vi "Stepper -- V3.vi"() -> ()   [LabVIEW 2018]
doc: "Use this template to build a producer/consumer design pattern with events to produce queue items. Use this design pattern instead of the User Interface Event Handler pattern for user interfaces when you want to execute code asynchronously in response to an event without slowing the user interface responsiveness."
uses:
  stepper motor state.ctl
  stepper graphics internal event.ctl
  stepper graphics action.ctl
  stepper graphics internal state.ctl
  stepper driver action.ctl
  publisher action.ctl
  slider action.ctl
  stepper driver -- BLM.vi
  stepper driver -- IMS.vi
panel:
  in  "Tab Control":enum32{"main", "init&stuff", "ignore"}(tab)
  in  "speed":i32=4003
  in  "stepper state":T1=enum."stopped"
  in  "set angle":dbl(slide)=-10.106382978723403 scale=-56.0..55.0 scale format="%^#6_6g"
  in  "XY Graph":cluster{dbl[], dbl[]}[](graph)=[{[-0.30000000000000004, -0.23550000000000004, -0.17100000000000004, -0.10650000000000004, -0.04200000000000004, 0.022499999999999964, 0.08699999999999997, 0.15149999999999997, 0.21599999999999997, 0.28049999999999997, 0.345, 0.4095, 0.474, 0.5385, 0.603, 0.6675, 0.732, 0.7965, 0.861, 0.9255], [0.0, 0.0, 0.0, 0.0, 0.0, 0.0, 0.0, 0.0, 0.0, 0.0, 0.0, 0.0, 0.0, 0.0, 0.0, 0.0, 0.0, 0.0, 0.0, 0.0]}, {[-0.29607463230851366, -0.23241858636218324, -0.1687625404158528, -0.10510649446952239, -0.04145044852319196, 0.02220559742313849, 0.08586164336946889, 0.14951768931579928, 0.21317373526212974, 0.2768297812084602, 0.34048582715479064, 0.404141873101121, 0.46779791904745144, 0.531453964993782, 0.5951100109401122, 0.6587660568864426, 0.7224221028327731, 0.7860781487791035, 0.849734194725434, 0.9133902406717644], [0.048371604308503874, 0.03797170938217554, 0.02757181445584721, 0.01717191952951888, 0.006772024603190548, -0.0036278703231377857, -0.014027765249466112, -0.024427660175794452, -0.03482755510212278, -0.045227450028451105, -0.055627344954779445, -0.06602723988110777, -0.0764271348074361, -0.08682702973376444, -0.09722692466009278, -0.10762681958642109, -0.11802671451274943, -0.12842660943907777, -0.13882650436540608, -0.14922639929173442]}, {[1.0, 0.9980267284282716, 0.9921147013144779, 0.9822872507286887, 0.9685831611286311, 0.9510565162951535, 0.9297764858882513, 0.9048270524660195, 0.8763066800438636, 0.8443279255020151, 0.8090169943749475, 0.7705132427757891, 0.7289686274214116, 0.6845471059286886, 0.6374239897486896, 0.587785252292473, 0.5358267949789965, 0.48175367410171516, 0.42577929156507266, 0.36812455268467786, 0.30901699437494745, 0.24868988716485474, 0.18738131458572452, 0.12533323356430426, 0.0627905195293133, -1.6081428723391245e-16, -0.0627905195293134, -0.12533323356430437, -0.18738131458572482, -0.24868988716485485, -0.30901699437494756, -0.368124552684678, -0.4257792915650727, -0.48175367410171543, -0.5358267949789969, -0.587785252292473, -0.6374239897486897, -0.6845471059286887, -0.7289686274214117, -0.7705132427757894, -0.8090169943749473, -0.8443279255020151, -0.8763066800438636, -0.9048270524660196, -0.9297764858882515, -0.9510565162951536, -0.9685831611286311, -0.9822872507286887, -0.9921147013144779, -0.9980267284282716, -1.0, -0.9980267284282716, -0.9921147013144779, -0.9822872507286886, -0.9685831611286311, -0.9510565162951535, -0.9297764858882512, -0.9048270524660195, -0.8763066800438635, -0.844327925502015, -0.8090169943749472, -0.770513242775789, -0.7289686274214116, -0.6845471059286886, -0.6374239897486895, -0.5877852522924732, -0.5358267949789963, -0.48175367410171527, -0.42577929156507216, -0.3681245526846778, -0.30901699437494756, -0.24868988716485443, -0.18738131458572463, -0.12533323356430373, -0.06279051952931321, -1.836909530733566e-16, 0.06279051952931372, 0.12533323356430423, 0.18738131458572513, 0.24868988716485493, 0.30901699437494723, 0.36812455268467825, 0.4257792915650726, 0.4817536741017157, 0.5358267949789968, 0.5877852522924737, 0.63742398974869, 0.6845471059286886, 0.7289686274214119, 0.7705132427757894, 0.8090169943749478, 0.8443279255020153, 0.8763066800438636, 0.9048270524660197, 0.9297764858882515, 0.9510565162951538, 0.9685831611286312, 0.9822872507286887, 0.9921147013144779, 0.9980267284282716], [0.0, 0.06279051952931337, 0.12533323356430426, 0.18738131458572463, 0.2486898871648548, 0.3090169943749474, 0.368124552684678, 0.4257792915650727, 0.4817536741017153, 0.5358267949789967, 0.5877852522924731, 0.6374239897486897, 0.6845471059286887, 0.7289686274214116, 0.7705132427757893, 0.8090169943749475, 0.8443279255020151, 0.8763066800438637, 0.9048270524660196, 0.9297764858882515, 0.9510565162951535, 0.9685831611286311, 0.9822872507286887, 0.9921147013144779, 0.9980267284282716, 1.0, 0.9980267284282716, 0.9921147013144778, 0.9822872507286886, 0.9685831611286311, 0.9510565162951535, 0.9297764858882513, 0.9048270524660195, 0.8763066800438635, 0.844327925502015, 0.8090169943749475, 0.7705132427757893, 0.7289686274214114, 0.6845471059286885, 0.6374239897486895, 0.5877852522924732, 0.5358267949789967, 0.4817536741017152, 0.4257792915650725, 0.36812455268467775, 0.3090169943749471, 0.24868988716485482, 0.18738131458572457, 0.1253332335643041, 0.06279051952931314, -3.216285744678249e-16, -0.06279051952931335, -0.12533323356430429, -0.18738131458572477, -0.24868988716485502, -0.30901699437494773, -0.3681245526846783, -0.42577929156507266, -0.4817536741017154, -0.5358267949789968, -0.5877852522924734, -0.63742398974869, -0.6845471059286887, -0.7289686274214116, -0.7705132427757894, -0.8090169943749473, -0.8443279255020153, -0.8763066800438636, -0.9048270524660198, -0.9297764858882515, -0.9510565162951535, -0.9685831611286312, -0.9822872507286887, -0.9921147013144779, -0.9980267284282716, -1.0, -0.9980267284282716, -0.9921147013144779, -0.9822872507286886, -0.9685831611286311, -0.9510565162951536, -0.9297764858882512, -0.9048270524660196, -0.8763066800438634, -0.844327925502015, -0.809016994374947, -0.770513242775789, -0.7289686274214116, -0.6845471059286883, -0.6374239897486896, -0.5877852522924726, -0.5358267949789963, -0.4817536741017153, -0.4257792915650722, -0.36812455268467786, -0.3090169943749468, -0.2486898871648545, -0.18738131458572468, -0.1253332335643038, -0.06279051952931326]}, {[0.1, 0.09980267284282716, 0.0992114701314478, 0.09822872507286888, 0.09685831611286311, 0.09510565162951536, 0.09297764858882514, 0.09048270524660196, 0.08763066800438636, 0.08443279255020152, 0.08090169943749476, 0.07705132427757892, 0.07289686274214116, 0.06845471059286887, 0.06374239897486897, 0.05877852522924731, 0.05358267949789966, 0.04817536741017152, 0.042577929156507266, 0.03681245526846779, 0.030901699437494747, 0.024868988716485477, 0.018738131458572452, 0.012533323356430426, 0.006279051952931331, -1.6081428723391246e-17, -0.0062790519529313405, -0.012533323356430438, -0.018738131458572484, -0.024868988716485487, -0.030901699437494757, -0.0368124552684678, -0.04257792915650727, -0.048175367410171546, -0.05358267949789969, -0.05877852522924731, -0.06374239897486898, -0.06845471059286888, -0.07289686274214117, -0.07705132427757894, -0.08090169943749474, -0.08443279255020152, -0.08763066800438636, -0.09048270524660196, -0.09297764858882515, -0.09510565162951537, -0.09685831611286311, -0.09822872507286888, -0.0992114701314478, -0.09980267284282716, -0.1, -0.09980267284282716, -0.0992114701314478, -0.09822872507286887, -0.09685831611286311, -0.09510565162951536, -0.09297764858882512, -0.09048270524660196, -0.08763066800438635, -0.0844327925502015, -0.08090169943749473, -0.07705132427757891, -0.07289686274214116, -0.06845471059286887, -0.06374239897486896, -0.05877852522924733, -0.05358267949789963, -0.04817536741017153, -0.04257792915650722, -0.036812455268467784, -0.030901699437494757, -0.024868988716485445, -0.018738131458572463, -0.012533323356430374, -0.006279051952931321, -1.836909530733566e-17, 0.006279051952931373, 0.012533323356430424, 0.018738131458572515, 0.024868988716485494, 0.030901699437494726, 0.036812455268467825, 0.042577929156507266, 0.048175367410171574, 0.05358267949789968, 0.05877852522924737, 0.063742398974869, 0.06845471059286887, 0.07289686274214119, 0.07705132427757894, 0.08090169943749478, 0.08443279255020153, 0.08763066800438636, 0.09048270524660197, 0.09297764858882515, 0.09510565162951538, 0.09685831611286312, 0.09822872507286888, 0.0992114701314478, 0.09980267284282716], [0.0, 0.006279051952931338, 0.012533323356430426, 0.018738131458572463, 0.02486898871648548, 0.03090169943749474, 0.0368124552684678, 0.04257792915650727, 0.04817536741017153, 0.05358267949789967, 0.058778525229247314, 0.06374239897486898, 0.06845471059286888, 0.07289686274214116, 0.07705132427757894, 0.08090169943749476, 0.08443279255020152, 0.08763066800438638, 0.09048270524660196, 0.09297764858882515, 0.09510565162951536, 0.09685831611286311, 0.09822872507286888, 0.0992114701314478, 0.09980267284282716, 0.1, 0.09980267284282716, 0.09921147013144778, 0.09822872507286887, 0.09685831611286311, 0.09510565162951536, 0.09297764858882514, 0.09048270524660196, 0.08763066800438635, 0.0844327925502015, 0.08090169943749476, 0.07705132427757894, 0.07289686274214115, 0.06845471059286885, 0.06374239897486896, 0.05877852522924733, 0.05358267949789967, 0.048175367410171525, 0.04257792915650725, 0.03681245526846778, 0.030901699437494712, 0.024868988716485484, 0.01873813145857246, 0.01253332335643041, 0.0062790519529313145, -3.216285744678249e-17, -0.006279051952931335, -0.01253332335643043, -0.018738131458572477, -0.024868988716485504, -0.030901699437494774, -0.03681245526846783, -0.042577929156507266, -0.04817536741017154, -0.05358267949789968, -0.05877852522924734, -0.063742398974869, -0.06845471059286888, -0.07289686274214116, -0.07705132427757894, -0.08090169943749474, -0.08443279255020153, -0.08763066800438636, -0.09048270524660199, -0.09297764858882515, -0.09510565162951536, -0.09685831611286312, -0.09822872507286888, -0.0992114701314478, -0.09980267284282716, -0.1, -0.09980267284282716, -0.0992114701314478, -0.09822872507286887, -0.09685831611286311, -0.09510565162951537, -0.09297764858882512, -0.09048270524660196, -0.08763066800438635, -0.0844327925502015, -0.0809016994374947, -0.07705132427757891, -0.07289686274214116, -0.06845471059286883, -0.06374239897486897, -0.05877852522924726, -0.05358267949789963, -0.04817536741017153, -0.042577929156507224, -0.03681245526846779, -0.03090169943749468, -0.02486898871648545, -0.01873813145857247, -0.012533323356430379, -0.006279051952931327]}, {[0.0, 0.0, 0.0, 0.0, 0.0, 0.0, 0.0, 0.0, 0.0, 0.0, 0.0, 0.0, 0.0, 0.0, 0.0, 0.0, 0.0, 0.0, 0.0, 0.0], [1.1, 1.135, 1.1700000000000002, 1.205, 1.24, 1.2750000000000001, 1.31, 1.345, 1.3800000000000001, 1.415, 1.4500000000000002, 1.485, 1.52, 1.5550000000000002, 1.59, 1.625, 1.6600000000000001, 1.695, 1.73, 1.7650000000000001]}, {[-0.09587131702242406, -0.09674287444990064, -0.09761443187737723, -0.0984859893048538, -0.0993575467323304, -0.10022910415980697, -0.10110066158728355, -0.10197221901476014, -0.10284377644223672, -0.10371533386971331, -0.10458689129718989, -0.10545844872466646, -0.10633000615214305, -0.10720156357961963, -0.10807312100709622, -0.1089446784345728, -0.10981623586204937, -0.11068779328952597, -0.11155935071700254, -0.11243090814447912], [1.0958141679009201, 1.1057761148818375, 1.115738061862755, 1.1257000088436726, 1.13566195582459, 1.1456239028055073, 1.1555858497864249, 1.1655477967673424, 1.1755097437482598, 1.1854716907291771, 1.1954336377100947, 1.2053955846910123, 1.2153575316719296, 1.225319478652847, 1.2352814256337645, 1.245243372614682, 1.2552053195955994, 1.2651672665765168, 1.2751292135574344, 1.285091160538352]}, {[-0.09587131702242406, -0.09674287444990064, -0.09761443187737723, -0.0984859893048538, -0.0993575467323304, -0.10022910415980697, -0.10110066158728355, -0.10197221901476014, -0.10284377644223672, -0.10371533386971331, -0.10458689129718989, -0.10545844872466646, -0.10633000615214305, -0.10720156357961963, -0.10807312100709622, -0.1089446784345728, -0.10981623586204937, -0.11068779328952597, -0.11155935071700254, -0.11243090814447912], [-1.0958141679009201, -1.1057761148818375, -1.115738061862755, -1.1257000088436726, -1.13566195582459, -1.1456239028055073, -1.1555858497864249, -1.1655477967673424, -1.1755097437482598, -1.1854716907291771, -1.1954336377100947, -1.2053955846910123, -1.2153575316719296, -1.225319478652847, -1.2352814256337645, -1.245243372614682, -1.2552053195955994, -1.2651672665765168, -1.2751292135574344, -1.285091160538352]}]
  out "cur angle":dbl(slide)=-9.278801002424245 scale=-95.0..95.0 scale format="%^#6_6g"
  in  "set step !":dbl(slide)=7372.340425531916 min=0.0 max=16000.0 scale=0.0..16500.0 scale format="%^#6_6g"
  out "cur step":dbl(slide)=7444.209386631578 scale=0.0..16500.0
  in  "Go!":bool
  in  "Stop!":bool
  in  "set speed!!":bool
  out "-- exit sync":bool
  in  "Instrument Address":refnum<visa-resource-name>="ASRL2::INSTR"
  in  "Set to zero!":bool
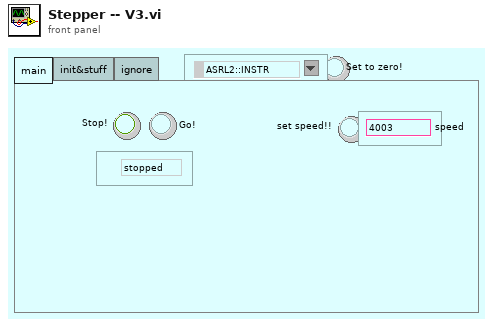
[diagram p1: front panel]
types:
  T1 = typedef "stepper motor state.ctl" = enum16{"moving", "stopped"}
  T2 = typedef "stepper driver action.ctl" = enum16{"go", "void", "stop", "check", "init", "sync", "set", "set speed", "--check status", "--check value"}
  T3 = typedef "stepper graphics internal state.ctl" = cluster{"set pos slider":refnum<vi>, "cur angle slider":refnum<vi>, "XY Graph":refnum<vi>, "set angle":dbl, "current angle":dbl, "set angle slider":refnum<vi>, "current pos... slider":refnum<vi>, "current pos":dbl, "set pos":dbl}
  T4 = typedef "stepper graphics action.ctl" = enum16{"--update circle", "set step slider moves", "cursor moves", "current pos changed", "init", "void", "--draw current lie", "--draw set line", "--move current step slider", "--move set step slider", "--draw limit lines", "check", "--move set angle slider", "--move current angle slider", "set angle slider moves", "--move cursor", "set set step", "set current step", "read"}
  T5 = typedef "stepper graphics internal event.ctl" = enum16{"set slider moves", "update scale", "exit", "current positon changed", "stop", "go", "set speed", "set to zero", "sync"}
  T6 = typedef "publisher action.ctl" = enum16{"set", "get"}
  T7 = typedef "slider action.ctl" = enum16{"check", "copy range", "set from value", "set from ratio", "set from slider", "read using other slider"}
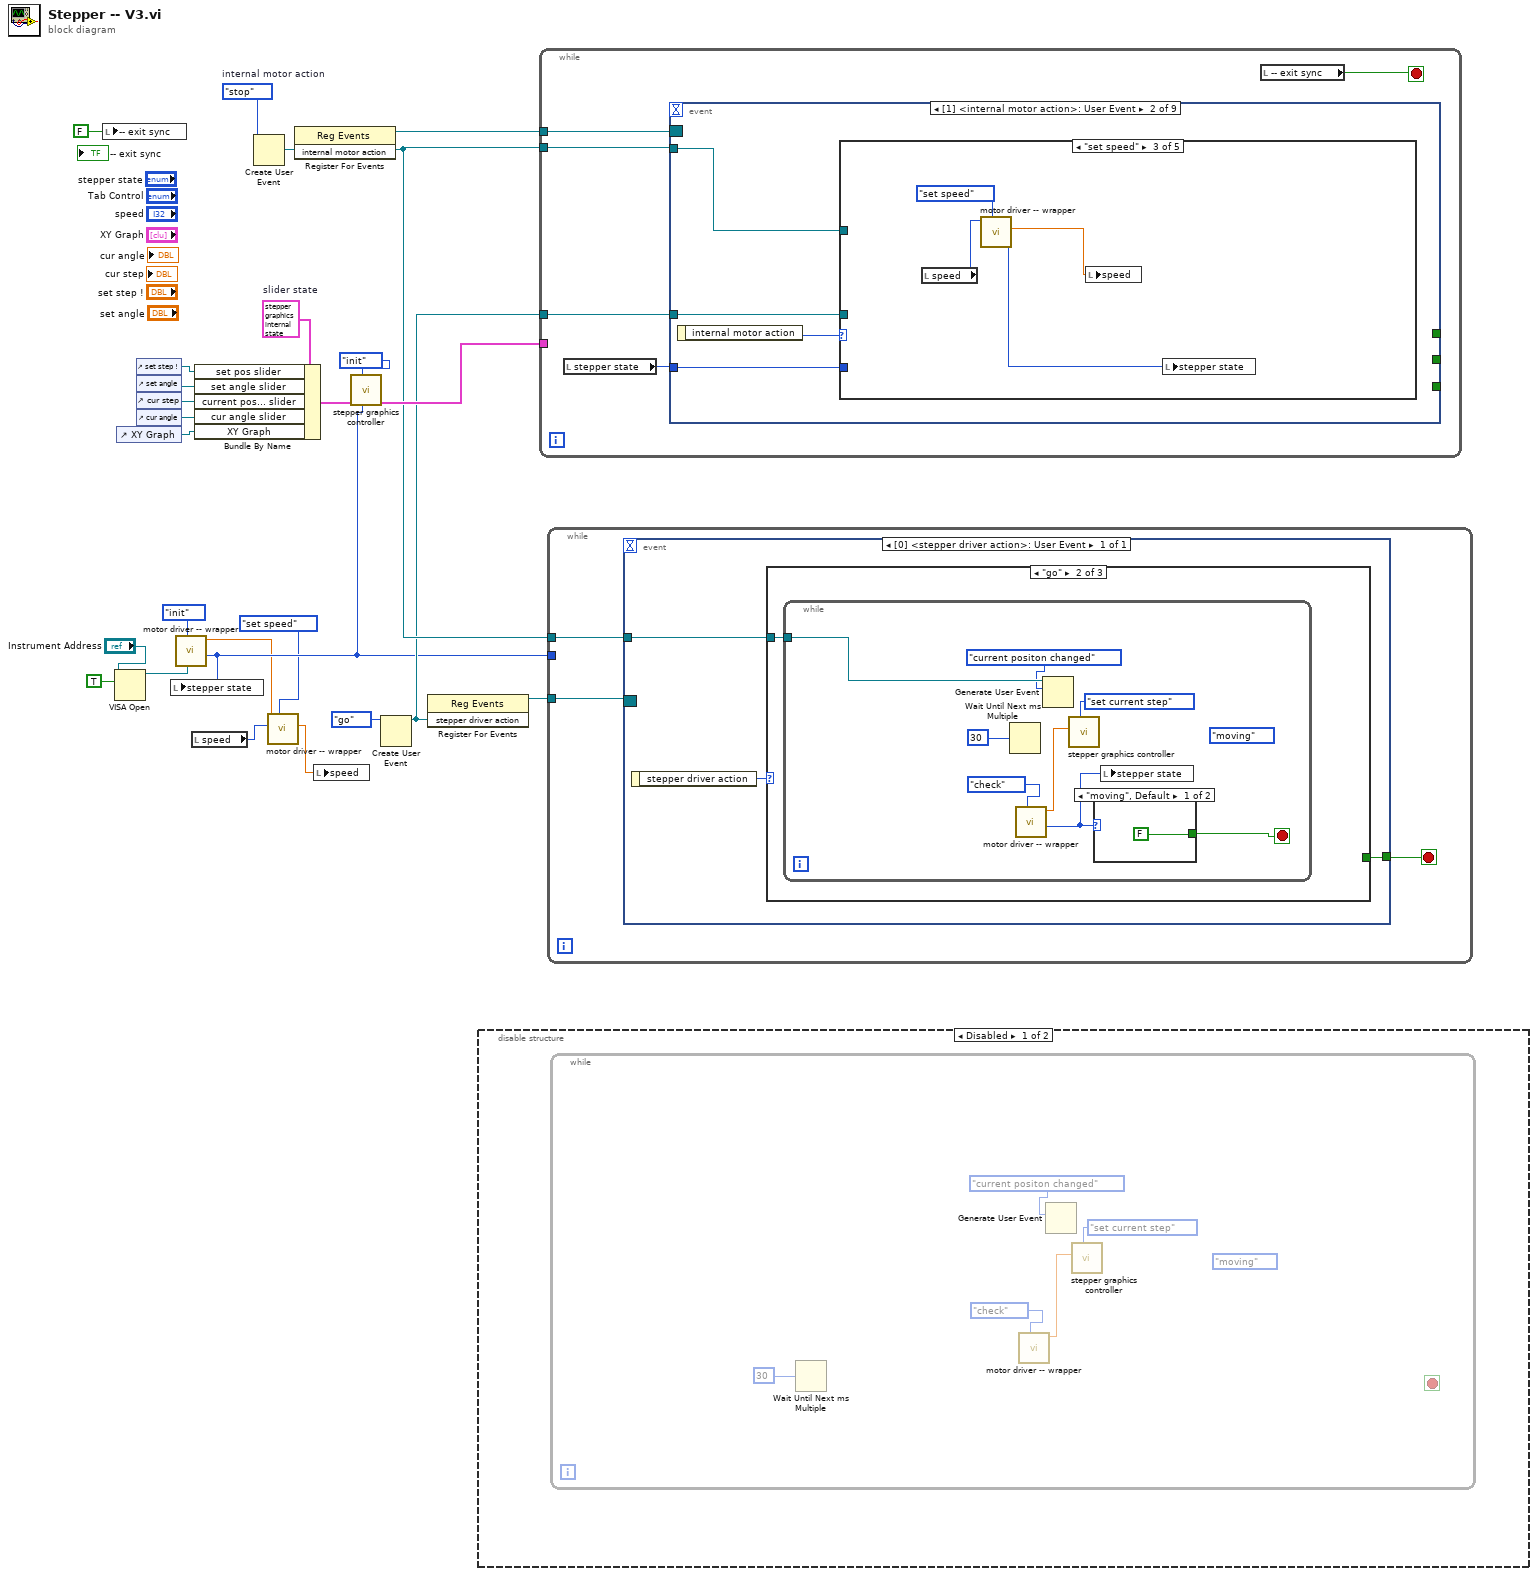
[diagram p0: block diagram]
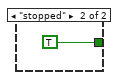
[diagram p4: hidden frame]
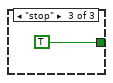
[diagram p5: hidden frame]
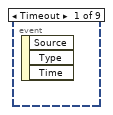
[diagram p6: hidden frame]
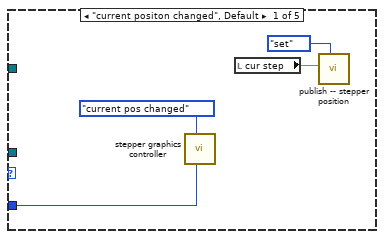
[diagram p7: hidden frame]
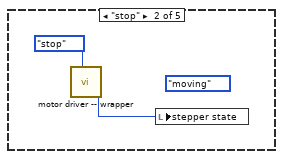
[diagram p8: hidden frame]
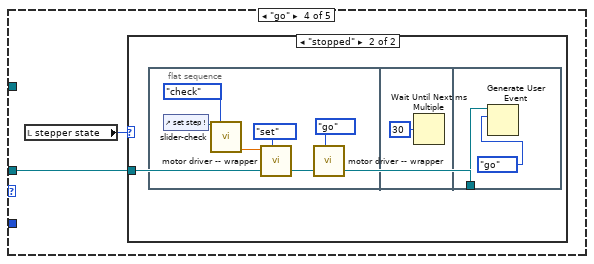
[diagram p9: hidden frame]
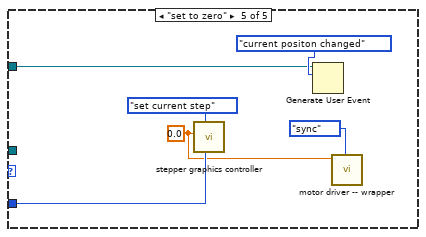
[diagram p11: hidden frame]
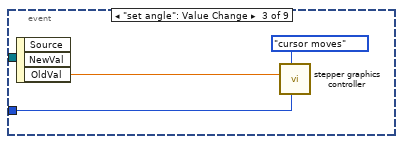
[diagram p12: hidden frame]
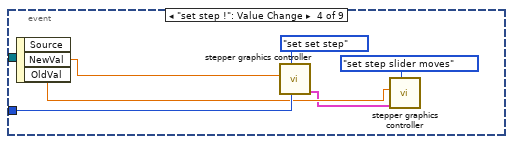
[diagram p13: hidden frame]
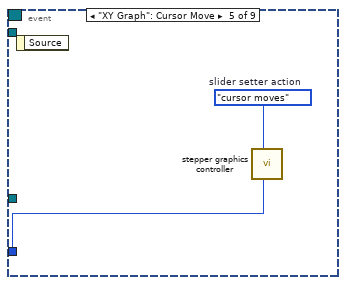
[diagram p14: hidden frame]
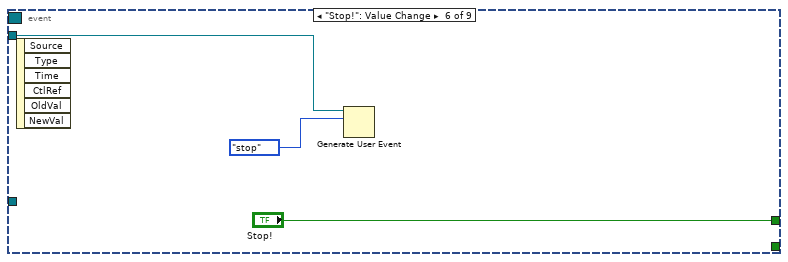
[diagram p15: hidden frame]
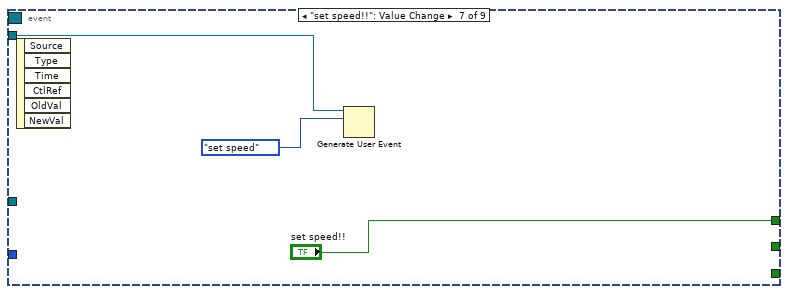
[diagram p16: hidden frame]
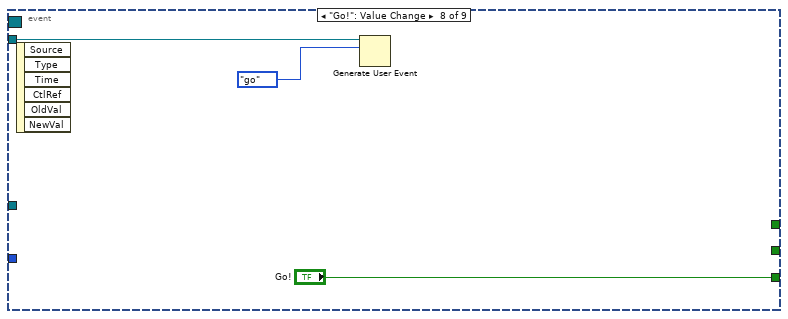
[diagram p17: hidden frame]
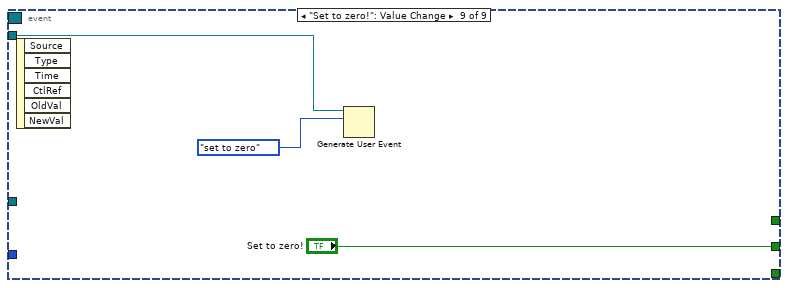
[diagram p18: hidden frame]
diagram:
  w20 = T3 {"set pos slider"=refnum, "cur angle slider"=refnum, "XY Graph"=refnum, "set angle"=0.0, "current angle"=0.0, "set angle slider"=refnum, "current pos... slider"=refnum, "current pos"=0.0, "set pos"=0.0}  # slider state
  w22 = stepper_graphics_internal_event."stop"  # internal motor action
  n1 = local write "-- exit sync"(FALSE ("-- exit  signal")) -> ()
  n2 = VISA Open(duplicate session (F)=TRUE, VISA resource name="Instrument Address") -> (VISA resource name=w1:refnum<visa-resource-name>)  [unwired: 3 in, 1 out]
  n3 = control-ref of="XY Graph"() -> (w19:refnum<vi>)
  n4 = control-ref of="set step !"() -> (w15:refnum<vi>)
  n5 = control-ref of="set angle"() -> (w16:refnum<vi>)
  n6 = control-ref of="cur step"() -> (w17:refnum<vi>)
  n7 = control-ref of="cur angle"() -> (w18:refnum<vi>)
  n8 = call "motor driver -- wrapper.vi"("Instrument Address"=w1, "stepper driver action"=stepper_driver_action."init") -> ("stepper motor state OUT"=w6:T1, "number OUT"=w2:dbl)  [unwired: 7 in, 1 out]
  n9 = local write "stepper state"(w6) -> ()
  n10 = local read "speed"() -> (w4:i32)
  n11 = Bundle By Name(cluster=w20, "set pos slider"=w15, "set angle slider"=w16, "current pos... slider"=w17, "cur angle slider"=w18, "XY Graph"=w19) -> (w14:T3)
  n12 = Create User Event(user event datatype=w22) -> (user event=w11:refnum<user-event>)  [unwired: 1 in, 1 out]
  n13 = call "motor driver -- wrapper.vi"("stepper driver action"=stepper_driver_action."set speed", "speed IN"=w4, "number IN"=w2) -> ("speed OUT"=w3:dbl)  [unwired: 6 in, 2 out]
  n14 = register-events(w11) -> (reference out=w23:refnum<event-registration>)  [unwired: 2 in, 1 out]
  n15 = local write "speed"(w3) -> ()
  n16 = call "stepper graphics controller.vi"("stepper motor state"=w6, "stepper graphics action"=stepper_graphics_action."init" ("slider setter action"), "stepper graphics internal state"=w14) -> ("stepper graphics internal state OUT"=w13:T3)  [unwired: 7 in, 1 out]
  n17 = Create User Event(user event datatype=stepper_driver_action."go" ("stepper driver action")) -> (user event=w7:refnum<user-event>)  [unwired: 1 in, 1 out]
  n18 = register-events(w7) -> (reference out=w9:refnum<event-registration>)  [unwired: 2 in, 1 out]
  n19 = disable-structure shown="Disabled" {
    frame Disabled {
      n20 = while {
        stop <- _ stop-if-true
        (unwired) stepper_motor_state."moving" ("stepper motor state OUT")
        n21 = Wait Until Next ms Multiple(millisecond multiple=u32 30) -> ()  [unwired: 1 out]
        n22 = call "motor driver -- wrapper.vi"("stepper driver action"=stepper_driver_action."check") -> ("number OUT"=w30:dbl)  [unwired: 8 in, 2 out]
        n23 = Generate User Event(event data cluster=stepper_graphics_internal_event."current positon changed" ("event data")) -> ()  [unwired: 3 in, 2 out]
        n24 = call "stepper graphics controller.vi"("stepper graphics action"=stepper_graphics_action."set current step" ("slider setter action"), "value"=w30) -> ()  [unwired: 8 in, 2 out]
      }
    }
    frame Enabled {
    }
  }
  n25 = while {
    tunnel: w23 -> [w35]
    tunnel: w11 -> [w34]
    tunnel: w13 -> [_]
    tunnel: w7 -> [w31]
    stop <- w32 stop-if-true
    n26 = local read "stepper state"() -> (w33:T1)
    n27 = event shown="[1] <internal motor action>: User Event" {
      selector: w35 -> [_ _ _ _ _ _ _ _ _]
      dyn-events: _ -> [_ _ _ _ _ _ _ _ _]
      timeout: _ -> [_ _ _ _ _ _ _ _ _]
      tunnel: w34 -> [_ w37 _ _ _ w79 w83 w86 w89]
      tunnel: w33 -> [_ w38 w67 w74 w76 _ _ _ _]
      tunnel: [_ _ _ _ _ "Stop!" "set speed!!" _ _] -> _
      tunnel: [_ _ _ _ _ _ _ "Go!" _] -> _
      tunnel: [_ _ _ _ _ _ _ _ "Set to zero!"] -> _
      tunnel: w31 -> [_ w36 _ _ _ _ _ _ _]
      event Timeout {
        n28 = event-data() -> ()  [unwired: 1 in, 3 out]
      }
      event User Event {
        n29 = event-data() -> ("internal motor action"=w39:T5)  [unwired: 1 in]
        n30 = case shown="\"set speed\"" w39 {
          tunnel: w38 -> [w40 _ _ _ w65]
          tunnel: w37 -> [_ _ _ _ w63]
          tunnel: w36 -> [_ _ _ w50 _]
          frame "current positon changed", Default {
            n31 = call "stepper graphics controller.vi"("stepper motor state"=w40, "stepper graphics action"=stepper_graphics_action."current pos changed" ("slider setter action")) -> ()  [unwired: 8 in, 2 out]
            n32 = local read "cur step"() -> (w42:dbl)
            n33 = call "publish -- stepper position.vi"("publisher action"=publisher_action."set", "stepper pos IN"=w42) -> ()  [unwired: 9 in, 1 out]
          }
          frame "stop" {
            (unwired) stepper_motor_state."moving" ("stepper motor state OUT")
            n34 = call "motor driver -- wrapper.vi"("stepper driver action"=stepper_driver_action."stop") -> ("stepper motor state OUT"=w44:T1)  [unwired: 8 in, 2 out]
            n35 = local write "stepper state"(w44) -> ()
          }
          frame "set speed" {
            n36 = local read "speed"() -> (w47:i32)
            n37 = call "motor driver -- wrapper.vi"("stepper driver action"=stepper_driver_action."set speed", "number IN"=w47) -> ("stepper motor state OUT"=w48:T1, "speed OUT"=w46:dbl)  [unwired: 7 in, 1 out]
            n38 = local write "speed"(w46) -> ()
            n39 = local write "stepper state"(w48) -> ()
          }
          frame "go" {
            n40 = local read "stepper state"() -> (w51:T1)
            n41 = case shown="\"stopped\"" w51 {
              tunnel: w50 -> [_ w52]
              frame "moving", Default {
              }
              frame "stopped" {
                n42 = flat-sequence {
                  tunnel: w52 -> [w60]
                  frame #0 {
                    n43 = control-ref of="set step !"() -> (w56:refnum<vi>)
                    n44 = call "slider-check.vi"("slider in"=w56, "slider action"=slider_action."check") -> ("value OUT"=w54:dbl)  [unwired: 9 in, 4 out]
                    n45 = call "motor driver -- wrapper.vi"("stepper driver action"=stepper_driver_action."set", "number IN"=w54) -> ()  [unwired: 7 in, 3 out]
                    n46 = call "motor driver -- wrapper.vi"("stepper driver action"=stepper_driver_action."go") -> ()  [unwired: 8 in, 3 out]
                  }
                  frame #1 {
                    n47 = Wait Until Next ms Multiple(millisecond multiple=u32 30) -> ()  [unwired: 1 out]
                  }
                  frame #2 {
                    n48 = Generate User Event(user event=w60, event data cluster=stepper_driver_action."go" ("event data")) -> ()  [unwired: 2 in, 2 out]
                  }
                }
              }
            }
          }
          frame "set to zero" {
            w61 = 0.0 ("value")
            n49 = call "stepper graphics controller.vi"("stepper motor state"=w65, "stepper graphics action"=stepper_graphics_action."set current step" ("slider setter action"), "value"=w61) -> ()  [unwired: 7 in, 2 out]
            n50 = Generate User Event(user event=w63, event data cluster=stepper_graphics_internal_event."current positon changed" ("event data")) -> ()  [unwired: 2 in, 2 out]
            n51 = call "motor driver -- wrapper.vi"("stepper driver action"=stepper_driver_action."sync", "number IN"=w61) -> ()  [unwired: 7 in, 3 out]
          }
        }
      }
      event "set angle": Value Change {
        n52 = event-data() -> ("OldVal"=w69:dbl)  [unwired: 1 in, 2 out]
        n53 = call "stepper graphics controller.vi"("stepper motor state"=w67, "stepper graphics action"=stepper_graphics_action."cursor moves" ("slider setter action"), "value"=w69) -> ()  [unwired: 7 in, 2 out]
      }
      event "set step !": Value Change {
        n54 = event-data() -> ("NewVal"=w72:dbl, "OldVal"=w71:dbl)  [unwired: 1 in, 1 out]
        n55 = call "stepper graphics controller.vi"("stepper motor state"=w74, "stepper graphics action"=stepper_graphics_action."set set step" ("slider setter action"), "value"=w72) -> ("stepper graphics internal state OUT"=w70:T3)  [unwired: 7 in, 1 out]
        n56 = call "stepper graphics controller.vi"("stepper graphics action"=stepper_graphics_action."set step slider moves" ("slider setter action"), "stepper graphics internal state"=w70, "value"=w71) -> ()  [unwired: 7 in, 2 out]
      }
      event "XY Graph": Cursor Move {
        w77 = stepper_graphics_action."cursor moves"  # slider setter action
        n57 = event-data() -> ()  [unwired: 1 in, 1 out]
        n58 = call "stepper graphics controller.vi"("stepper motor state"=w76, "stepper graphics action"=w77) -> ()  [unwired: 8 in, 2 out]
      }
      event "Stop!": Value Change {
        n59 = event-data() -> ()  [unwired: 1 in, 6 out]
        n60 = Generate User Event(user event=w79, event data cluster=stepper_graphics_internal_event."stop" ("event data")) -> ()  [unwired: 2 in, 2 out]
      }
      event "set speed!!": Value Change {
        n61 = event-data() -> ()  [unwired: 1 in, 6 out]
        n62 = Generate User Event(user event=w83, event data cluster=stepper_graphics_internal_event."set speed" ("event data")) -> ()  [unwired: 2 in, 2 out]
      }
      event "Go!": Value Change {
        n63 = event-data() -> ()  [unwired: 1 in, 6 out]
        n64 = Generate User Event(user event=w86, event data cluster=stepper_graphics_internal_event."go" ("event data")) -> ()  [unwired: 2 in, 2 out]
      }
      event "Set to zero!": Value Change {
        n65 = event-data() -> ()  [unwired: 1 in, 6 out]
        n66 = Generate User Event(user event=w89, event data cluster=stepper_graphics_internal_event."set to zero" ("event data")) -> ()  [unwired: 2 in, 2 out]
      }
    }
    n67 = local read "-- exit sync"() -> (w32:bool)
  }
  n68 = while {
    tunnel: w11 -> [w92]
    tunnel: w9 -> [w91]
    tunnel: w6 -> [_]
    stop <- w90 stop-if-true
    n69 = event shown="[0] <stepper driver action>: User Event" {
      selector: w91 -> [_]
      dyn-events: _ -> [_]
      timeout: _ -> [_]
      tunnel: w92 -> [w95]
      tunnel: [w93] -> w90
      event User Event {
        n70 = event-data() -> ("stepper driver action"=w94:T2)  [unwired: 1 in]
        n71 = case shown="\"go\"" w94 {
          tunnel: w95 -> [_ w96 _]
          tunnel: [_ _ TRUE] -> w93
          frame "void", Default {
          }
          frame "go" {
            n72 = while {
              tunnel: w96 -> [w104]
              stop <- w98 stop-if-true
              (unwired) stepper_motor_state."moving" ("stepper motor state OUT")
              # "This loop is a consumer loop."
              n73 = Wait Until Next ms Multiple(millisecond multiple=u32 30) -> ()  [unwired: 1 out]
              n74 = call "motor driver -- wrapper.vi"("stepper driver action"=stepper_driver_action."check") -> ("stepper motor state OUT"=w97:T1, "number OUT"=w103:dbl)  [unwired: 8 in, 1 out]
              n75 = Generate User Event(user event=w104, event data cluster=stepper_graphics_internal_event."current positon changed" ("event data")) -> ()  [unwired: 2 in, 2 out]
              n76 = call "stepper graphics controller.vi"("stepper graphics action"=stepper_graphics_action."set current step" ("slider setter action"), "value"=w103) -> ()  [unwired: 8 in, 2 out]
              n77 = case shown="\"moving\", Default" w97 {
                tunnel: [FALSE TRUE] -> w98
                frame "moving", Default {
                }
                frame "stopped" {
                }
              }
              n78 = local write "stepper state"(w97) -> ()
            }
          }
          frame "stop" {
          }
        }
      }
    }
  }
